vi "AdjustDisplay.vi"(8 "error in (no error)":errorcluster caption="错误输入（无错误）", 11 "DigitalDisplay 输入":refnum<class "DigitalDisplay.lvclass">) -> (0 "error out":errorcluster caption="错误输出", 3 "DigitalDisplay 输出":refnum<class "DigitalDisplay.lvclass">)   [LabVIEW 2018, in "DataDisplay.lvlib" / "DigitalDisplay.lvclass"]
uses:
  DigitalDisplay.lvclass
  DigitalDisplay.lvclass/DigitalDisplay.ctl
  SubVI/DD_Parameter.vi
  DataDisplay.lvlib
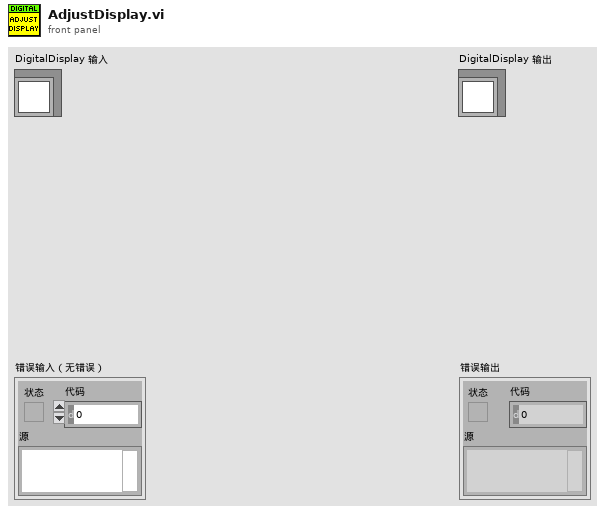
[diagram p1: front panel]
types:
  T1 = typedef "LVRectTypeDef.ctl" = cluster{"Left":i16, "Top":i16, "Right":i16, "Bottom":i16}
  T2 = typedef "DataDisplay.lvlib/DD_ChannelInfo.ctl" = cluster{"名称":string, "单位":string, "数据类型":enum16{"Real", "Int"}, "趋势线":enum16{"N/A", "X", "Y"}}
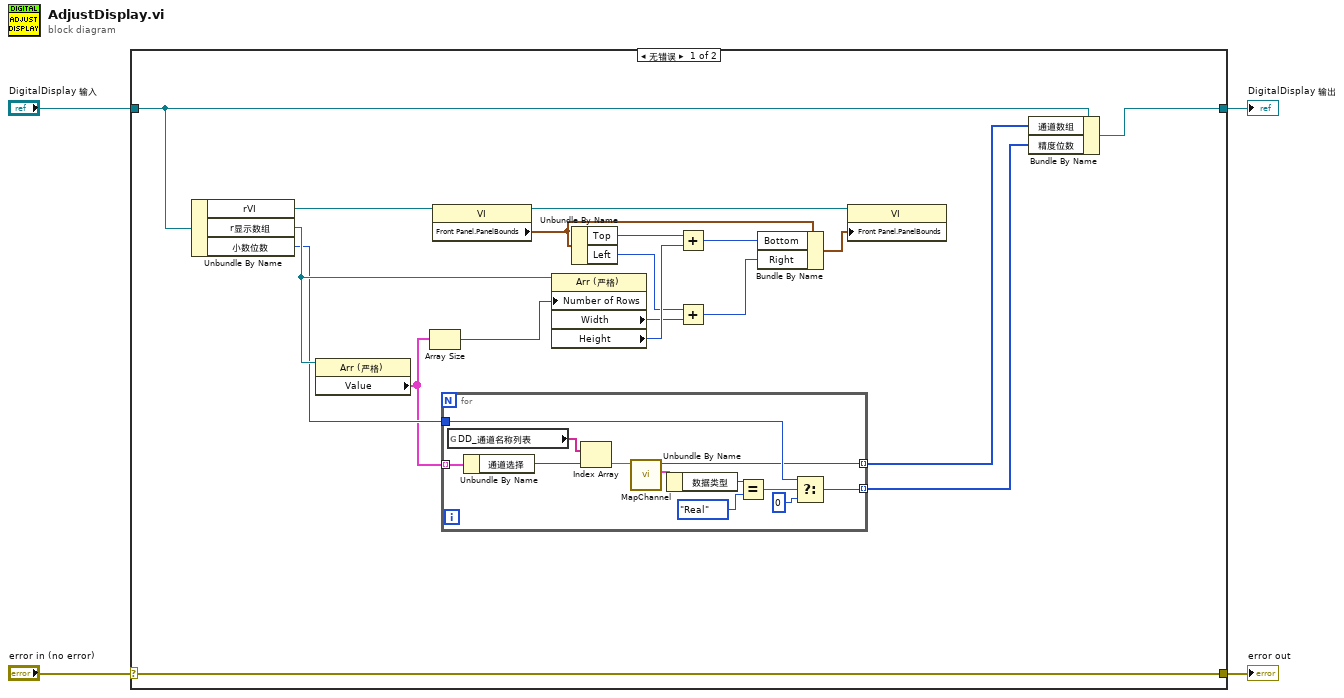
[diagram p0: block diagram]
diagram:
  n1 = case shown="无错误" "error in (no error)" {
    selector: "error in (no error)" -> [w23 w37]
    tunnel: [w23 w37] -> w3
    tunnel: [w7 w36] -> w1
    tunnel: "DigitalDisplay 输入" -> [w12 w36]
    frame No Error {
      n2 = Unbundle By Name(w12) -> ("rVI"=w11:refnum<vi>, "r显示数组"=w10:refnum<vi>, "小数位数"=w9:u8)
      n3 = property class="Arr (严格)"(reference=w10) -> ("Value"=w8:cluster{"通道选择":u16, "数值":string}[])  [unwired: 1 in, 2 out]
      n4 = Array Size(array=w8) -> (size(s)=w17:i32)
      n5 = property class="VI"(reference=w11) -> (reference out=w21:refnum<vi>, "Front Panel.PanelBounds"=w14:T1)  [unwired: 1 in, 1 out]
      n6 = for {
        tunnel: w8 -> [w35] mode=indexing
        tunnel: [w32] -> w6 mode=indexing
        tunnel: w9 -> [w28]
        tunnel: [w26] -> w5 mode=indexing
        n7 = global read "DD_Parameter.vi" "DD_通道名称列表"() -> (w30:string[])
        n8 = Unbundle By Name(w35) -> ("通道选择"=w29:u16)
        n9 = Index Array(array=w30, index=w29) -> (element=w27:string)
        n10 = call "MapChannel.vi"("通道名称"=w27) -> ("通道信息"=w25:T2, "索引"=w26:i32)  [unwired: 9 in]
        n11 = Unbundle By Name(w25) -> ("数据类型"=w24:enum16{"Real", "Int"})
        n12 = Equal?(x=w24, y=enum16{"Real", "Int"}."Real") -> (x = y?=w34:bool)
        n13 = Select(t=w28, s=w34, f=0) -> (s? t:f=w32:i32)
      }
      n14 = property class="Arr (严格)"(reference=w10, "Number of Rows"=w17) -> ("Width"=w19:u32, "Height"=w22:u32)  [unwired: 1 in, 2 out]
      n15 = Unbundle By Name(w14) -> ("Top"=w13:i16, "Left"=w18:i16)
      n16 = Add(x=w13, y=w22) -> (x+y=w15:u32)
      n17 = Add(x=w18, y=w19) -> (x+y=w20:u32)
      n18 = Bundle By Name(cluster=w14, "Bottom"=w15, "Right"=w20) -> (w16:T1)
      n19 = property class="VI"(reference=w21, "Front Panel.PanelBounds"=w16) -> ()  [unwired: 1 in, 2 out]
      n20 = Bundle By Name(cluster=w12, "通道数组"=w5, "精度位数"=w6) -> (w7:refnum<class "DigitalDisplay.lvclass">)
    }
    frame Error {
    }
  }
  "error out" <- w3
  "DigitalDisplay 输出" <- w1
